vi "Online_Station.vi"(8 "error in (no error)":errorcluster, 11 "Main":T1={"Tite"="", "Base path"=path "", "Table"=[], "Stations"=[], "Shield Array"=[], "UPHs"=[], "VISA"={"VISA"="", "baud rate"=9600, "data bits"=8, "parity"=enum."None", "stop bits"=10, "flow control"=0}, "Path"={"roof"=path "", "Config"=path "", "Png"=path ""}, "Ctr"={"DB Dispaly"=refnum, "Error Table"=refnum, "Display"=refnum, "Login"=refnum, "Exit"=refnum, "FTT_Submit"=refnum}, "Login"={"User"="", "Grade"=""}, "information"={"cause"="", "Type"=enum."Inform", "code"=0, "Suroce"="", "Status"=FALSE}, "Local DB"={"Connstr"="", "Database"={"Constr"={"Driver"="", "Server"="", "User"="", "Pwd"="", "Database"=""}, "conn ref"=refnum, "State"=FALSE}}, "Remote DB"={"Connstr"="", "Database"={"Constr"={"Driver"="", "Server"="", "User"="", "Pwd"="", "Database"=""}, "conn ref"=refnum, "State"=FALSE}}, "FTT TV"="", "ExchangeTime"=0, "NVH"="", "EOL Path"=path ""} {"VISA"."flow control" items=["None", "XON/XOFF", "RTS/CTS", "XON/XOFF & RTS/CTS", "DTR/DSR", "XON/XOFF & DTR/DSR"]; "VISA"."stop bits" items=["1.0"=10, "1.5"=15, "2.0"=20]}) -> (0 "error out":errorcluster)   [LabVIEW 2014]
uses:
  Type'def/Online_Table.ctl
  <vilib>/ptbypt/NI_PtbyPt.lvlib
  Simatic S7/Function/Read/Read Sigle Data/Read Sigle String.vi
  <vilib>/addons/database/Connection.llb/Conn ObjectReference.ctl
  <vilib>/addons/database/NI_Database_API.lvlib
  Simatic S7/Function/Read/Read Sigle Data/Read Sigle Bool.vi
  Type'def/UPH Config.ctl
  VISA/Ctr/VISA Ctr.ctl
  Type'def/Main Ctr Ref.ctl
  Type'def/User Login.ctl
  Type'def/MainCtr.ctl
  Database/Ctr/Constr.ctl
  Database/Ctr/Conneect State.ctl
panel:
  out "Previous Event 2":string
  out "Previous Event":string
  in  "Test":bool
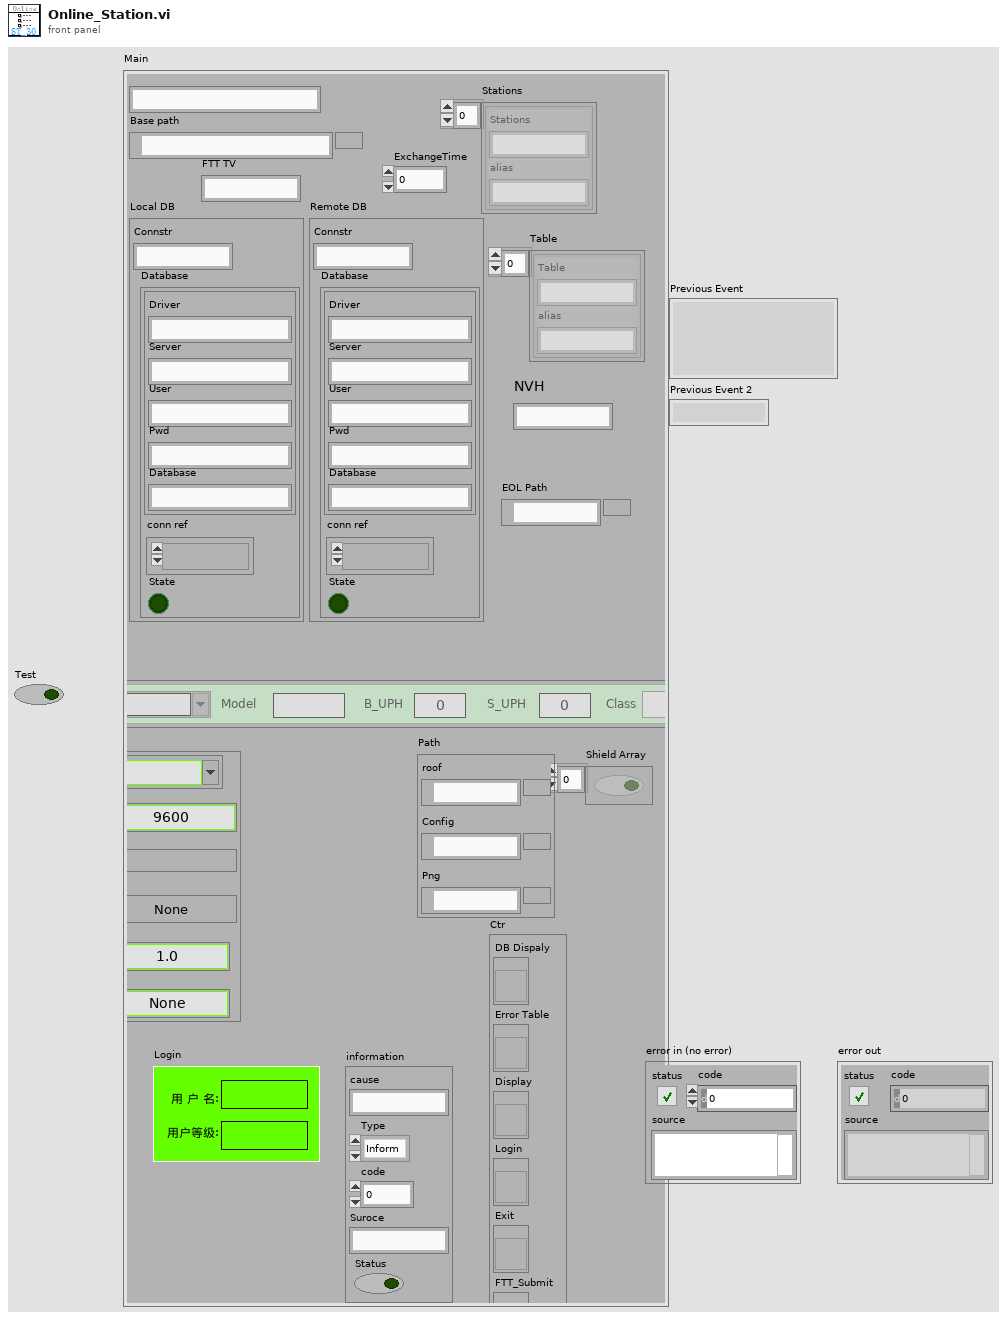
[diagram p1: front panel]
types:
  T1 = typedef "MainCtr.ctl" = cluster{"Tite":string, "Base path":path, "Table":cluster{"Table":string, "alias":string}[], "Stations":cluster{"Stations":string, "alias":string}[], "Shield Array":bool[], "UPHs":T2[], "VISA":T3, "Path":cluster{"roof":path, "Config":path, "Png":path}, "Ctr":T4, "Login":T5, "information":cluster{"cause":string, "Type":enum16{"Inform", "Warning", "Alarm"}, "code":i32, "Suroce":string, "Status":bool}, "Local DB":cluster{"Connstr":string, "Database":T6}, "Remote DB":cluster{"Connstr":string, "Database":T6}, "FTT TV":string, "ExchangeTime":i32, "NVH":string, "EOL Path":path}
  T2 = typedef "UPH Config.ctl" = cluster{"Line_No":string, "Model":string, "B_UPH ":i16, "S_UPH  ":i16, "Class":enum16{"Big", "Small"}}
  T3 = typedef "VISA Ctr.ctl" = cluster{"VISA":refnum<visa-resource-name>, "baud rate":u32, "data bits":u16, "parity":enum16{"None", "Odd", "Even", "Mark", "Space"}, "stop bits":u16, "flow control":u16}
  T4 = typedef "Main Ctr Ref.ctl" = cluster{"DB Dispaly":refnum<vi>, "Error Table":refnum<vi>, "Display":refnum<vi>, "Login":refnum<vi>, "Exit":refnum<vi>, "FTT_Submit":refnum<vi>}
  T5 = typedef "User Login.ctl" = cluster{"User":string, "Grade":string}
  T6 = typedef "Conneect State.ctl" = cluster{"Constr":T7, "conn ref":T8, "State":bool}
  T7 = typedef "Constr.ctl" = cluster{"Driver":string, "Server":string, "User":string, "Pwd":string, "Database":string}
  T8 = typedef "NI_Database_API.lvlib/Conn ObjectReference.ctl" = refnum<k1>
  T9 = cluster{"cause":string, "Type":enum16{"Inform", "Warning", "Alarm"}, "code":i32, "Suroce":string, "Status":bool}
  T10 = typedef "Online_Table.ctl" = cluster{"SN":string, "Frame":string, "Station":string, "Model":string, "Color":string, "OnTime":timestamp, "OutTime":timestamp, "Repaired":i32, "OnRepair":bool, "Pstate":string}
  T11 = cluster{"Main ":T1, "Online_Table":T10, "information":cluster{"cause":string, "Type":enum16{"Inform", "Warning", "Alarm"}, "code":i32, "Suroce":string, "Status":bool}, "ns":dbl}
  T12 = typedef "FTT Display Type.ctl" = cluster{"Line.No":string, "Model":string, "Color":string, "UPH":dbl, "Plan":dbl, "Target Rate":dbl, "Target ":dbl, "Actual":dbl, "FTT":dbl, "FTT Rate":dbl, "Repaired":dbl, "Reject":dbl, "Ouline":dbl, "Line State":string}
  T13 = cluster{"Display":T12, "Class":enum16{"Big", "Small"}}
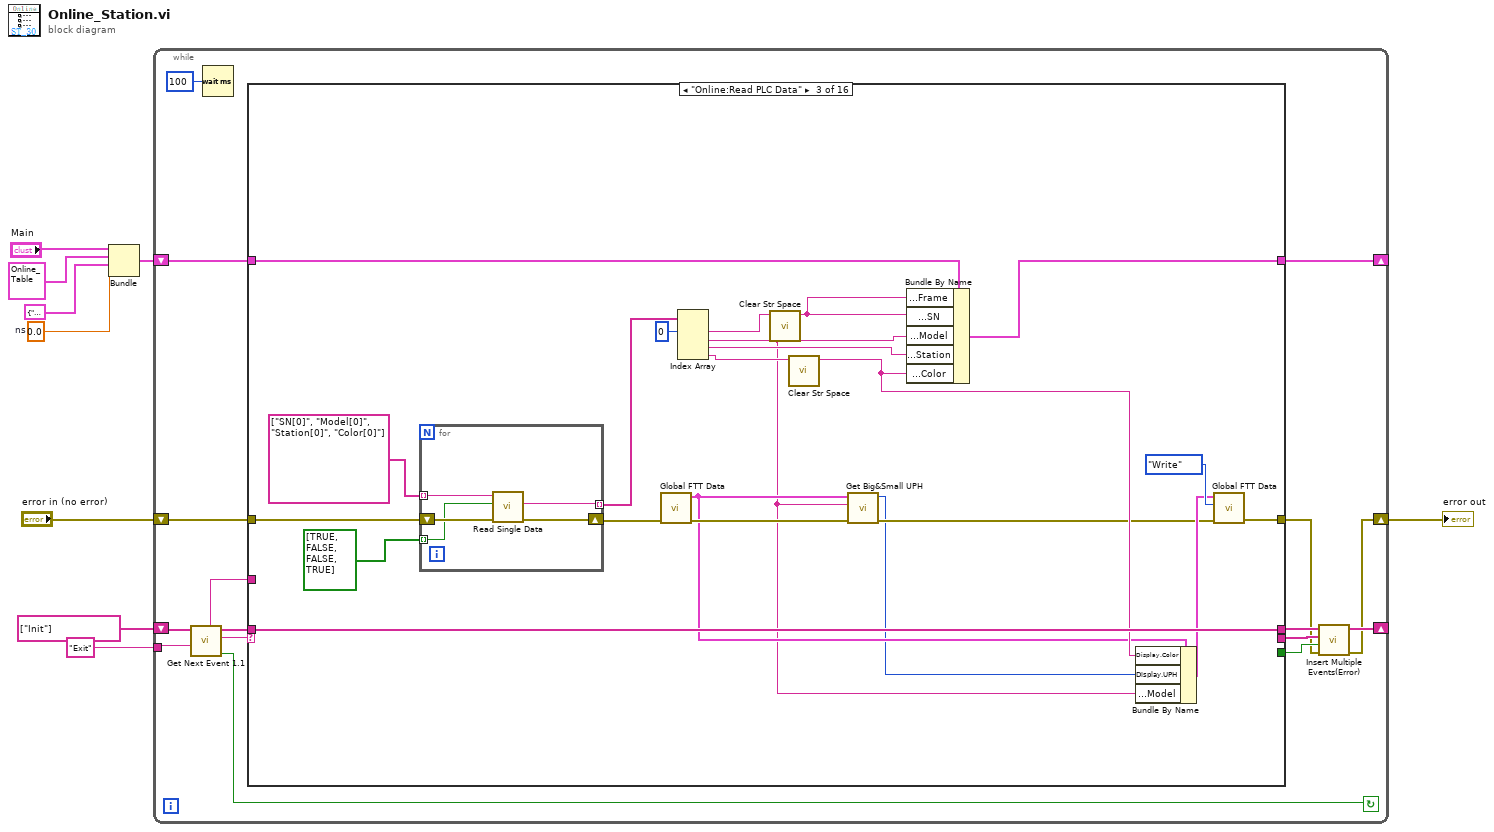
[diagram p0: block diagram]
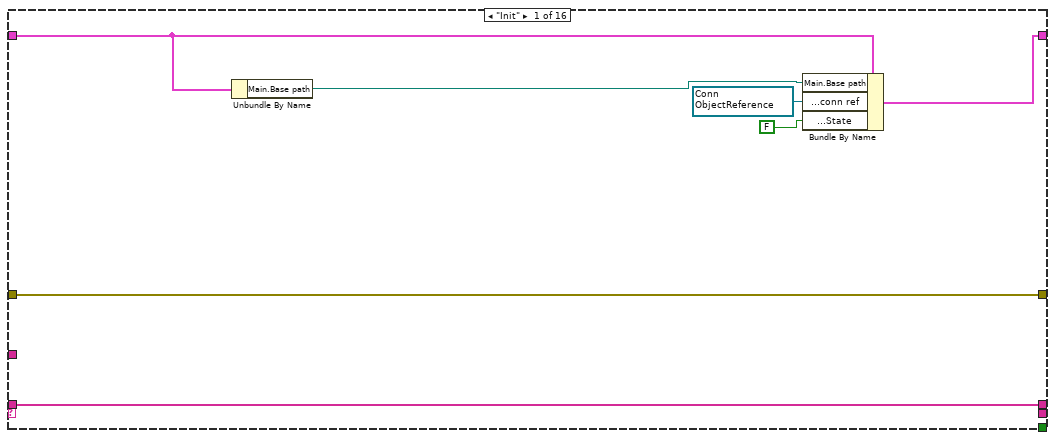
[diagram p2: hidden frame]
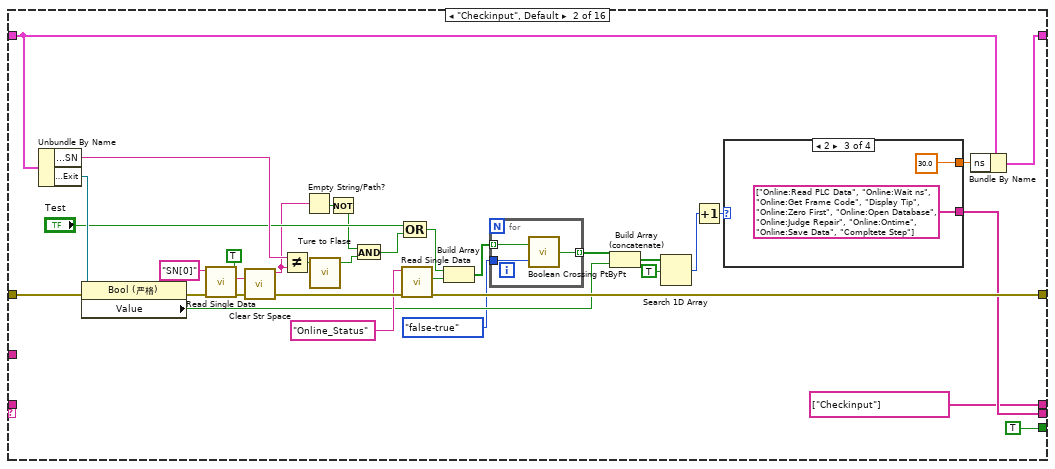
[diagram p3: hidden frame]
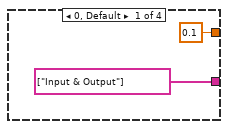
[diagram p4: hidden frame]
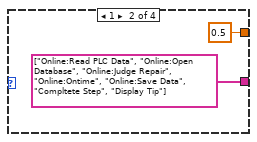
[diagram p5: hidden frame]
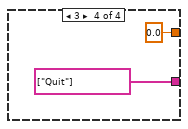
[diagram p6: hidden frame]
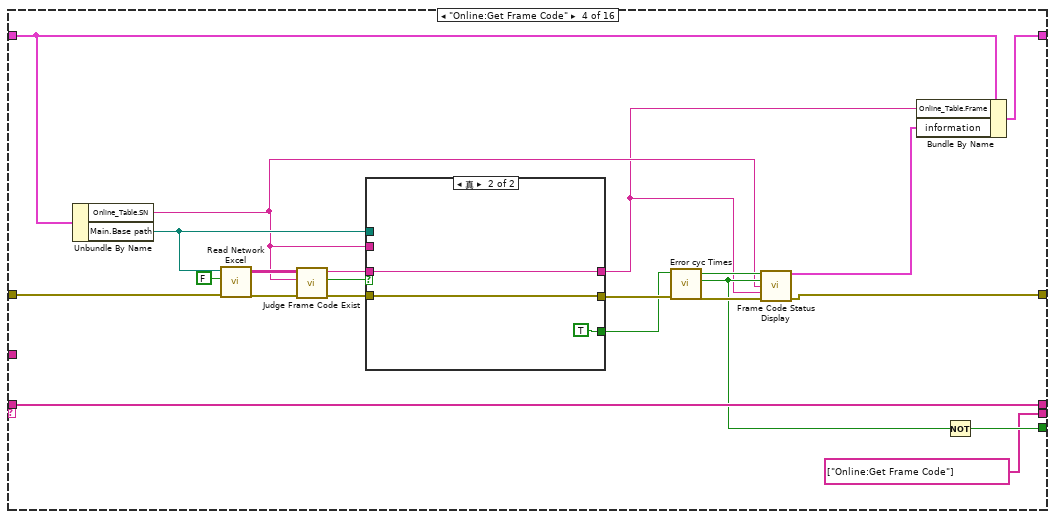
[diagram p7: hidden frame]
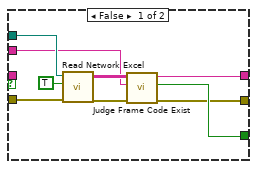
[diagram p8: hidden frame]
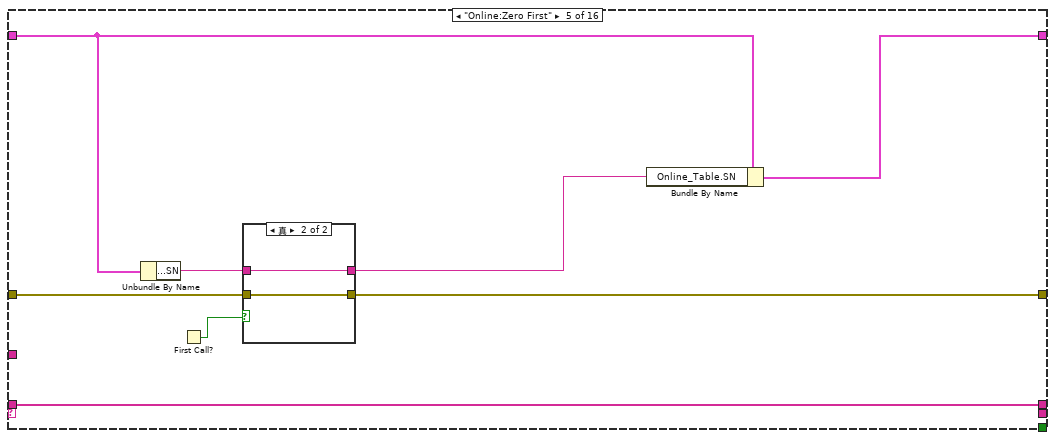
[diagram p9: hidden frame]
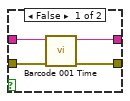
[diagram p10: hidden frame]
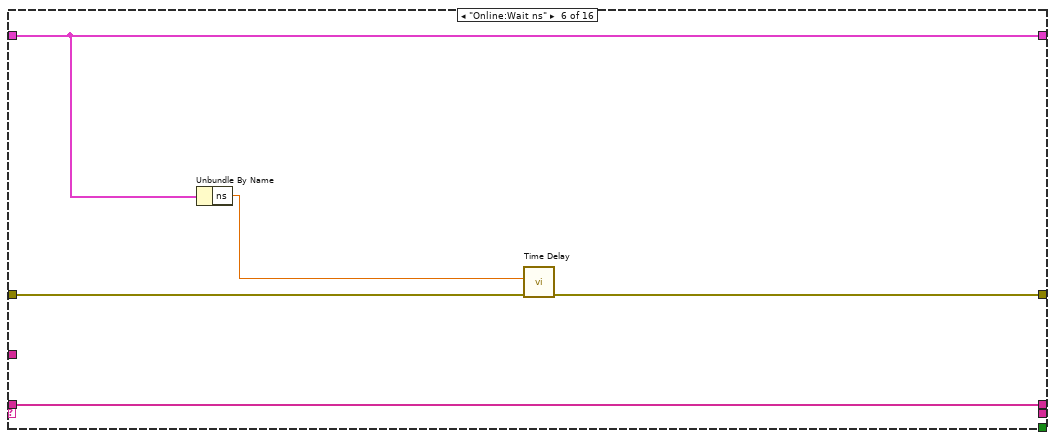
[diagram p11: hidden frame]
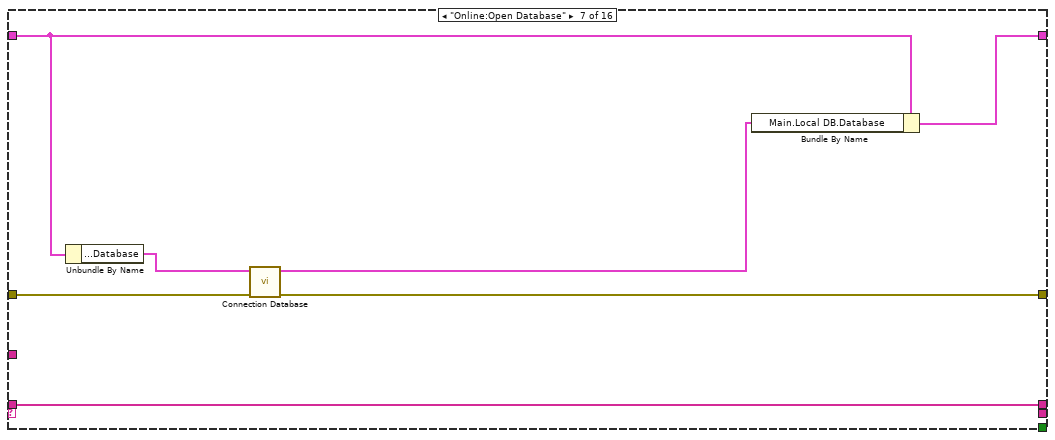
[diagram p12: hidden frame]
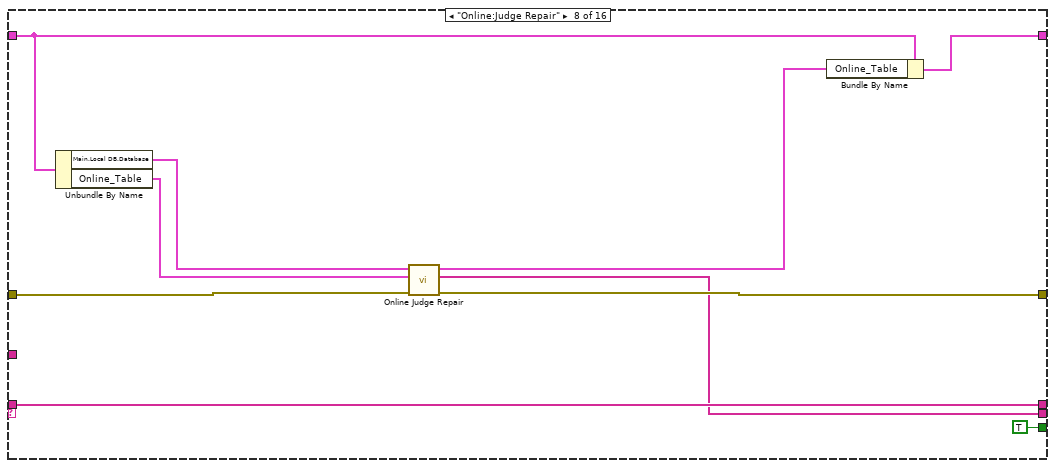
[diagram p13: hidden frame]
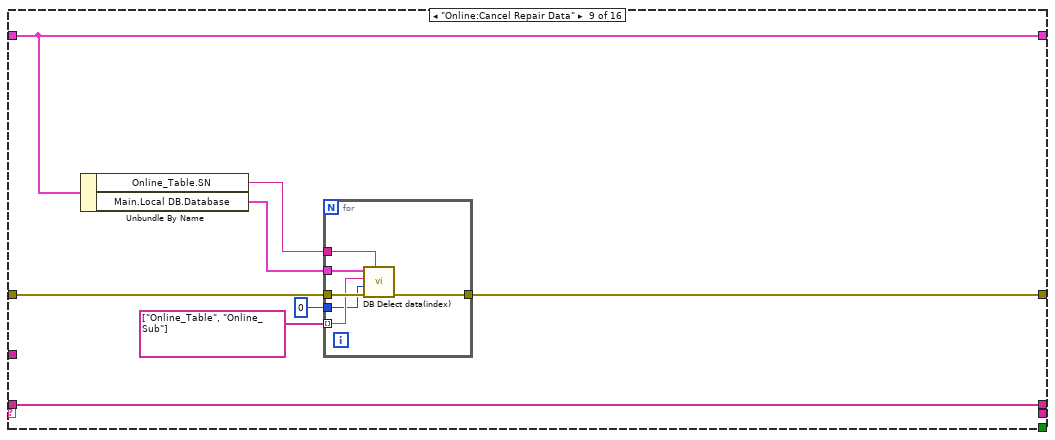
[diagram p14: hidden frame]
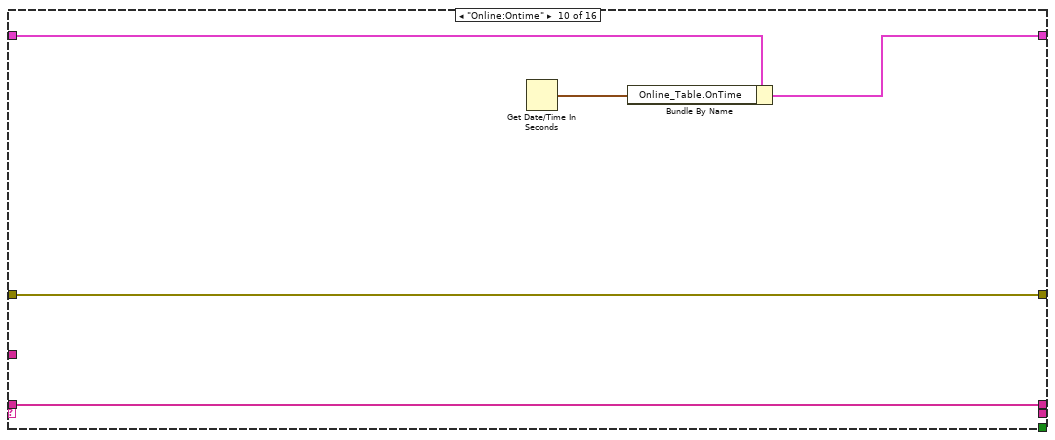
[diagram p15: hidden frame]
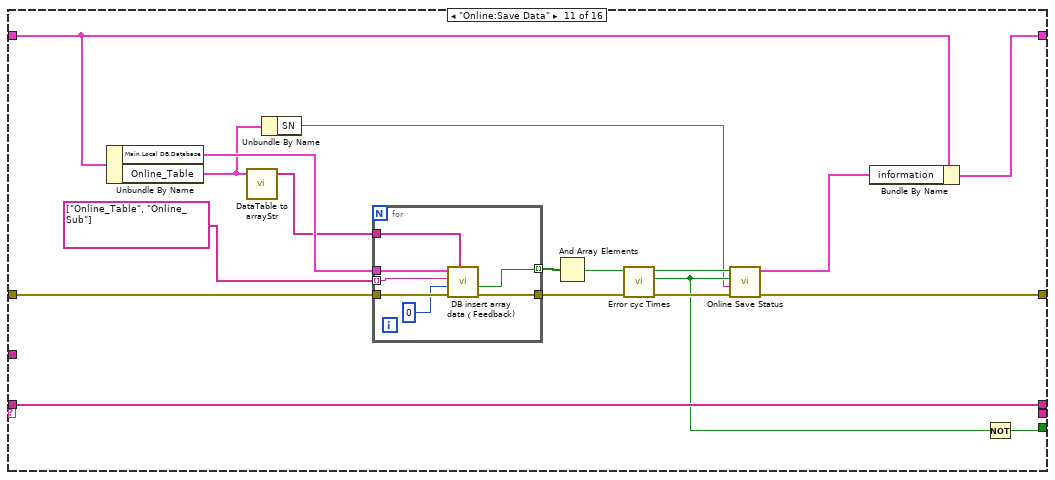
[diagram p16: hidden frame]
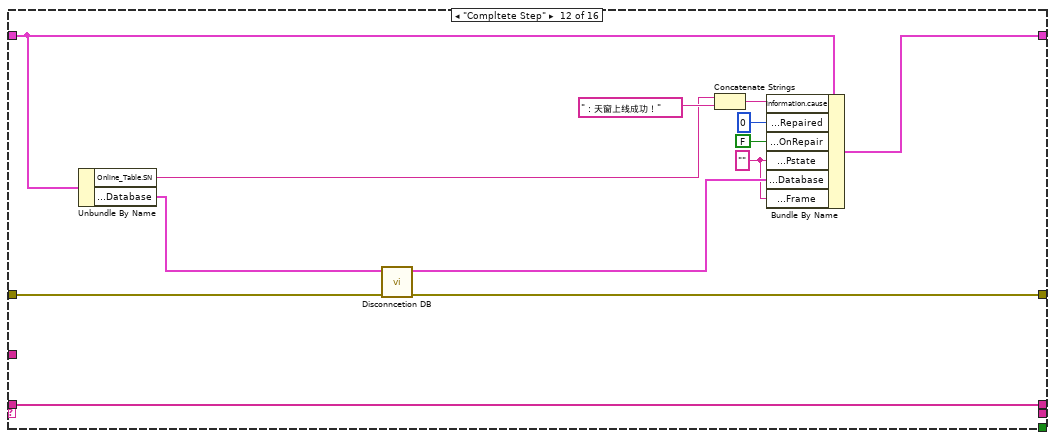
[diagram p17: hidden frame]
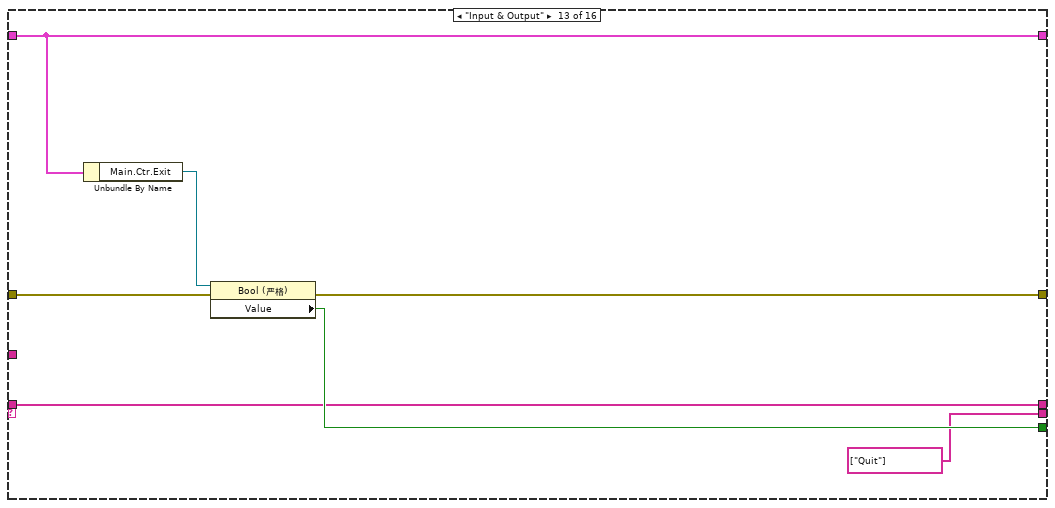
[diagram p18: hidden frame]
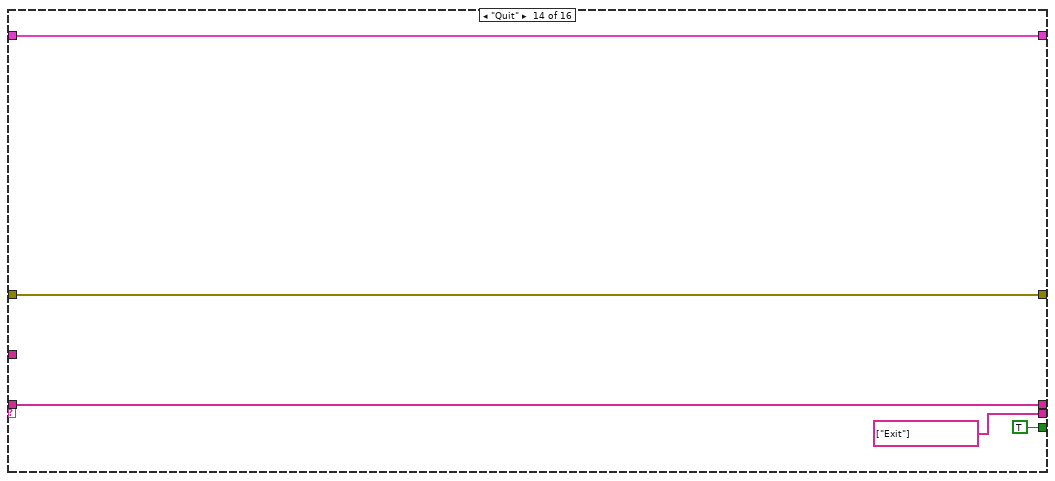
[diagram p19: hidden frame]
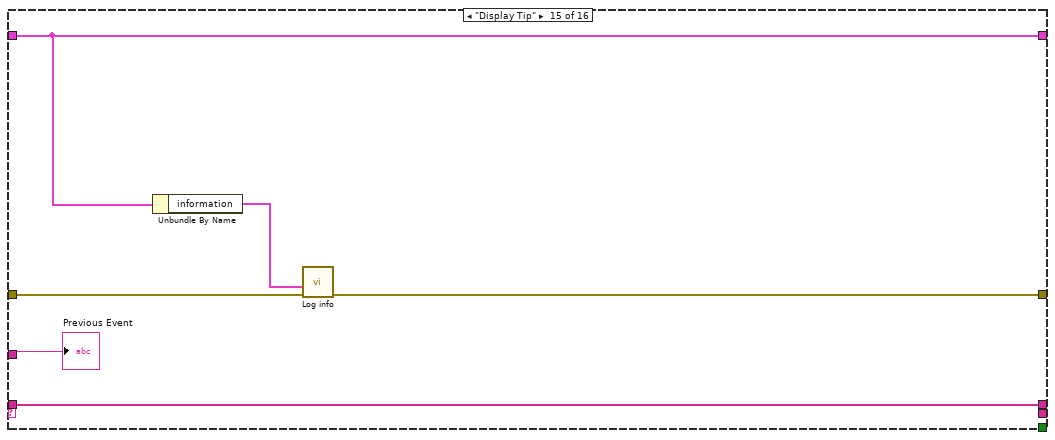
[diagram p20: hidden frame]
diagram:
  w1 = 0.0  # ns
  n1 = Bundle("Main"="Main", "Online_Table"=T10 {"SN"="", "Frame"="", "Station"="", "Model"="", "Color"="", "OnTime"=timestamp(0 s since 1904-01-01), "OutTime"=timestamp(0 s since 1904-01-01), "Repaired"=0, "OnRepair"=FALSE, "Pstate"=""}, "information"=T9 {"cause"="", "Type"=enum."Inform", "code"=0, "Suroce"="", "Status"=FALSE}, "ns"=w1) -> (w6:T11)  [unwired: 1 in]
  n2 = while {
    tunnel: "Exit" ("Exit Event") -> [w22]
    shift-right: [w18] -> _
    shift-left: string[] ["Init"] -> [w23]
    shift-right: [w12] -> w3
    shift-left: "error in (no error)" -> [w21]
    shift-right: [w14] -> _
    shift-left: w6 -> [w19]
    stop <- w24 continue-if-true
    n3 = call "Get Next Event 1.1.vi"("Exit Event"=w22, "event queue in"=w23) -> ("Condition (Exit:F)"=w24:bool, "next event"=w25:string, "event queue out"=w20:string[], "Previous Event"=w10:string)  [unwired: 6 in]
    n4 = Wait (ms)(milliseconds to wait=u32 100) -> ()  [unwired: 1 out]
    n5 = case shown="\"Online:Read PLC Data\"" w25 {
      tunnel: w21 -> [w31 w64 w98 w124 w144 w156 w160 w172 w179 w188 w209 w226 w236 w241 w248 w252]
      tunnel: w20 -> [w32 _ w94 w125 w142 w154 w163 w173 w181 w190 w210 w230 w232 w240 w244 _]
      tunnel: w19 -> [w29 w42 w96 w118 w141 w153 w162 w169 w180 w189 w194 w224 w237 w242 w246 w257]
      tunnel: [w31 w56 w88 w105 w143 w155 w158 w166 w174 w188 w200 w225 w234 w241 w247 w258] -> w13
      tunnel: [w32 string[] ["Checkinput"] w94 w125 w142 w154 w163 w173 w181 w190 w210 w230 w232 w240 w244 string[] ["Checkinput"]] -> w17
      tunnel: [_ TRUE ("Insert all? (T)") _ w113 _ _ _ TRUE ("Insert all? (T)") _ _ w202 _ w233 TRUE ("Insert all? (T)") _ FALSE ("Insert all? (T)")] -> w16
      tunnel: [_ w49 _ string[] ["Online:Get Frame Code"] _ _ _ w165 _ _ _ _ string[] ["Quit"] string[] ["Exit"] _ _] -> w15
      tunnel: [w30 w41 w95 w117 w140 w153 w161 w168 w180 w191 w193 w229 w237 w242 w246 w257] -> w14
      tunnel: w10 -> [_ _ _ _ _ _ _ _ _ _ _ _ _ _ w243 w250]
      frame "Init" {
        w27 = T8 refnum items=["Connection"] ("conn refer.conn ref")
        n6 = Unbundle By Name(w29) -> ("Main.Base path"=w28:path)
        n7 = Bundle By Name(cluster=w29, "Main.Base path"=w28, "Main.Local DB.Database.conn ref"=w27, "Main.Local DB.Database.State"=FALSE ("conn refer.State")) -> (w30:T11)
      }
      frame "Checkinput", Default {
        n8 = Unbundle By Name(w42) -> ("Online_Table.SN"=w61:string, "Main.Ctr.Exit"=w65:refnum<vi>)
        n9 = property class="Bool (严格)"(reference=w65, error in=w64) -> (error out=w63:errorcluster, "Value"=w55:bool)  [unwired: 1 out]
        n10 = call-poly "Read Single Data.vi"("error in (no error)"=w63, "Char/Str"=TRUE, "Tags"="SN[0]") -> ("error out"=w59:errorcluster, "Data Byte"=w39:string)  [unwired: 6 in, 1 out]
        n11 = call "Clear Str Space.vi"("SN"=w39) -> ("字符串"=w37:string)  [unwired: 10 in]
        n12 = Not Equal?(x=w61, y=w37) -> (x != y?=w60:bool)
        n13 = Empty String/Path?(string/path=w37) -> (empty?=w36:bool)
        n14 = call "Ture to Flase.vi"("in"=w60) -> ("Out"=w35:bool)  [unwired: 4 in]
        n15 = Not(x=w36) -> (.not. x?=w34:bool)
        n16 = And(x=w34, y=w35) -> (x .and. y?=w33:bool)
        n17 = call-poly "Read Single Data.vi"("error in (no error)"=w59, "Tags"="Online_Status") -> ("error out"=w56:errorcluster, "Boolean"=w46:bool)  [unwired: 7 in, 1 out]
        n18 = Compound Arithmetic op=OR("Test", w33) -> (w47:bool)
        n19 = Build Array(w47, w46) -> (w45:bool[])
        n20 = for {
          tunnel: w45 -> [w68] mode=indexing
          tunnel: enum16{"either", "false-true", "true-false"}."false-true" ("direction") -> [w67]
          tunnel: [w66] -> w43 mode=indexing
          n21 = call <vilib>:"Boolean Crossing PtByPt.vi"("direction"=w67, "input"=w68) -> ("crossing"=w66:bool)  [unwired: 1 in]
        }
        n22 = Build Array (concatenate)(w43, w55) -> (w54:bool[])
        n23 = Search 1D Array(1D array=w54, element=TRUE) -> (index of element=w52:i32)  [unwired: 1 in]
        n24 = Increment(x=w52) -> (x+1=w50:i32)
        n25 = case shown="2" w50 {
          tunnel: [string[] ["Input & Output"] string[] ["Online:Read PLC Data", "Online:Open Database", "Online:Judge Repair", "Online:Ontime", "Online:Save Data", "Compltete Step", "Display Tip"] string[] ["Online:Read PLC Data", "Online:Wait ns", "Online:Get Frame Code", "Display Tip", "Online:Zero First", "Online:Open Database", "Online:Judge Repair", "Online:Ontime", "Online:Save Data", "Compltete Step"] string[] ["Quit"]] -> w49
          tunnel: [0.1 0.5 30.0 0.0] -> w40
          frame 0, Default {
          }
          frame 1 {
          }
          frame 2 {
          }
          frame 3 {
          }
        }
        n26 = Bundle By Name(cluster=w42, "ns"=w40) -> (w41:T11)
      }
      frame "Online:Read PLC Data" {
        n27 = for {
          shift-right: [w102] -> w90
          shift-left: w98 -> [w103]
          tunnel: string[] ["SN[0]", "Model[0]", "Station[0]", "Color[0]"] -> [w101] mode=indexing
          tunnel: [w100] -> w93 mode=indexing
          tunnel: bool[] [TRUE, FALSE, FALSE, TRUE] -> [w99] mode=indexing
          n28 = call-poly "Read Single Data.vi"("error in (no error)"=w103, "Char/Str"=w99, "Tags"=w101) -> ("error out"=w102:errorcluster, "Data Byte"=w100:string)  [unwired: 6 in, 1 out]
        }
        n29 = call "Global FTT Data.vi"("error in (no error)"=w90) -> ("error out"=w81:errorcluster, "Cluster"=w80:T13)  [unwired: 9 in]
        n30 = Index Array(array=w93, index #1=0 ("index")) -> (element #1=w85:string, element #2=w79:string, element #3=w92:string, element #4=w83:string)  [unwired: 3 in]
        n31 = call "Clear Str Space.vi"("SN"=w85) -> ("字符串"=w84:string)  [unwired: 10 in]
        n32 = call "Clear Str Space.vi"("SN"=w83) -> ("字符串"=w82:string)  [unwired: 10 in]
        n33 = call "Get Big&Small UPH.vi"("error in (no error)"=w81, "Model"=w79, "Cluster"=w80) -> ("error out"=w78:errorcluster, "UPH"=w77:i16)  [unwired: 7 in]
        n34 = Bundle By Name(cluster=w96, "Online_Table.Frame"=w84, "Online_Table.SN"=w84, "Online_Table.Model"=w79, "Online_Table.Station"=w92, "Online_Table.Color"=w82) -> (w95:T11)
        n35 = Bundle By Name(cluster=w80, "Display.Color"=w82, "Display.UPH"=w77, "Display.Model"=w79) -> (w87:T13)
        n36 = call "Global FTT Data.vi"("error in (no error)"=w78, "Mode"=enum16{"Read", "Write"}."Write", "Display"=w87) -> ("error out"=w88:errorcluster)  [unwired: 7 in, 1 out]
      }
      frame "Online:Get Frame Code" {
        n37 = Unbundle By Name(w118) -> ("Online_Table.SN"=w108:string, "Main.Base path"=w116:path)
        n38 = call "Read Network Excel.vi"("error in (no error)"=w124, "T/Y"=FALSE, "Base Path"=w116) -> ("error out"=w123:errorcluster, "2DA_Str"=w122:string[][])  [unwired: 7 in]
        n39 = call "Judge Frame Code Exist.vi"("error in (no error)"=w123, "Online_Table.SN"=w108, "2DA_Str"=w122) -> ("error out"=w121:errorcluster, "Status"=w120:bool, "Frame Code"=w119:string)  [unwired: 6 in]
        n40 = case shown="真" w120 {
          tunnel: w121 -> [w133 w135]
          tunnel: w119 -> [_ w137]
          tunnel: [w127 w137] -> w107
          tunnel: w116 -> [w132 _]
          tunnel: w108 -> [w129 _]
          tunnel: [w128 TRUE ("Status")] -> w114
          tunnel: [w126 w135] -> w115
          frame False {
            n41 = call "Read Network Excel.vi"("error in (no error)"=w133, "T/Y"=TRUE, "Base Path"=w132) -> ("error out"=w134:errorcluster, "2DA_Str"=w130:string[][])  [unwired: 7 in]
            n42 = call "Judge Frame Code Exist.vi"("error in (no error)"=w134, "Online_Table.SN"=w129, "2DA_Str"=w130) -> ("error out"=w126:errorcluster, "Status"=w128:bool, "Frame Code"=w127:string)  [unwired: 6 in]
          }
          frame True {
          }
        }
        n43 = call "Error cyc Times.vi"("error in (no error)"=w115, "Status in"=w114) -> ("error out"=w111:errorcluster, "Cys Status"=w109:bool, "Status out"=w110:bool)  [unwired: 6 in, 1 out]
        n44 = call "Frame Code Status Display.vi"("Status"=w110, "Complete"=w109, "SN"=w108, "Frame"=w107, "error in (no error)"=w111) -> ("information"=w106:T9, "error out"=w105:errorcluster)  [unwired: 9 in]
        n45 = Bundle By Name(cluster=w118, "Online_Table.Frame"=w107, "information"=w106) -> (w117:T11)
        n46 = Not(x=w109) -> (.not. x?=w113:bool)
      }
      frame "Online:Zero First" {
        n47 = Unbundle By Name(w141) -> ("Online_Table.SN"=w145:string)
        n48 = First Call?() -> (First Call?: T/F=w138:bool)
        n49 = case shown="真" w138 {
          tunnel: w145 -> [w149 w150]
          tunnel: w144 -> [w148 w151]
          tunnel: [w147 w151] -> w143
          tunnel: [w146 w150] -> w139
          frame False {
            n50 = call "Barcode 001 Time.vi"("error in (no error)"=w148, "Code"=w149) -> ("error out"=w147:errorcluster, "Code out"=w146:string)  [unwired: 8 in]
          }
          frame True {
          }
        }
        n51 = Bundle By Name(cluster=w141, "Online_Table.SN"=w139) -> (w140:T11)
      }
      frame "Online:Wait ns" {
        n52 = Unbundle By Name(w153) -> ("ns"=w152:dbl)
        n53 = call "Time Delay"("error in (no error)"=w156, "Delay Time (s)"=w152) -> ("error out"=w155:errorcluster)  [unwired: 9 in]
      }
      frame "Online:Open Database" {
        n54 = Unbundle By Name(w162) -> ("Main.Local DB.Database"=w159:T6)
        n55 = call "Connection Database.vi"("error in (no error)"=w160, "Connncet State"=w159) -> ("error out"=w158:errorcluster, "Connncet State out"=w157:T6)  [unwired: 8 in]
        n56 = Bundle By Name(cluster=w162, "Main.Local DB.Database"=w157) -> (w161:T11)
      }
      frame "Online:Judge Repair" {
        n57 = Unbundle By Name(w169) -> ("Main.Local DB.Database"=w171:T6, "Online_Table"=w170:T10)
        n58 = call "Online Judge Repair.vi"("error in (no error)"=w172, "Online_Table"=w170, "conn refer"=w171) -> ("error out"=w166:errorcluster, "Steps"=w165:string[], "Online_Table out"=w167:T10)  [unwired: 6 in]
        n59 = Bundle By Name(cluster=w169, "Online_Table"=w167) -> (w168:T11)
      }
      frame "Online:Cancel Repair Data" {
        n60 = Unbundle By Name(w180) -> ("Online_Table.SN"=w175:string, "Main.Local DB.Database"=w178:T6)
        n61 = for {
          tunnel: w179 -> [w187]
          tunnel: w178 -> [w186]
          tunnel: string[] ["Online_Table", "Online_Sub"] -> [w185] mode=indexing
          tunnel: 0 ("index") -> [w184]
          tunnel: w175 -> [w183]
          tunnel: [w182] -> w174
          n62 = call "DB Delect data(index).vi"("code"=w183, "error in (no error)"=w187, "index"=w184, "table"=w185, "Connncet State"=w186) -> ("error out"=w182:errorcluster)  [unwired: 4 in, 2 out]
        }
      }
      frame "Online:Ontime" {
        n63 = Get Date/Time In Seconds() -> (seconds since 1Jan1904=w192:timestamp)
        n64 = Bundle By Name(cluster=w189, "Online_Table.OnTime"=w192) -> (w191:T11)
      }
      frame "Online:Save Data" {
        n65 = Unbundle By Name(w194) -> ("Main.Local DB.Database"=w208:T6, "Online_Table"=w197:T10)
        n66 = call "DataTable to arrayStr.vi"("Online_Table"=w197) -> ("appended array"=w206:string[])  [unwired: 4 in]
        n67 = Unbundle By Name(w197) -> ("SN"=w196:string)
        n68 = for {
          tunnel: w209 -> [w217]
          tunnel: w208 -> [w216]
          tunnel: string[] ["Online_Table", "Online_Sub"] -> [w215] mode=indexing
          tunnel: [w213] -> w204
          tunnel: w206 -> [w212]
          tunnel: [w211] -> w205 mode=indexing
          n69 = call "DB insert array data（Feedback).vi"("Data"=w212, "error in (no error)"=w217, "index"=0, "table"=w215, "Connncet State"=w216) -> ("error out"=w213:errorcluster, "state"=w211:bool)  [unwired: 4 in, 1 out]
        }
        n70 = And Array Elements(Boolean array=w205) -> (logical AND=w203:bool)
        n71 = call "Error cyc Times.vi"("error in (no error)"=w204, "Status in"=w203) -> ("error out"=w201:errorcluster, "Cys Status"=w198:bool, "Status out"=w199:bool)  [unwired: 6 in, 1 out]
        n72 = call "Online Save Status.vi"("error in (no error)"=w201, "SN"=w196, "Complete"=w198, "Status"=w199) -> ("error out"=w200:errorcluster, "information"=w195:T9)  [unwired: 6 in]
        n73 = Bundle By Name(cluster=w194, "information"=w195) -> (w193:T11)
        n74 = Not(x=w198) -> (.not. x?=w202:bool)
      }
      frame "Compltete Step" {
        w218 = "" ("Online_Table.Pstate")
        n75 = Unbundle By Name(w224) -> ("Online_Table.SN"=w220:string, "Main.Local DB.Database"=w223:T6)
        n76 = call "Disconncetion DB.vi"("error in (no error)"=w226, "Connncet State"=w223) -> ("error out"=w225:errorcluster, "Connect State"=w219:T6)  [unwired: 8 in]
        n77 = Concatenate Strings(w220, "：天窗上线成功！" ("information.cause")) -> (w222:string)
        n78 = Bundle By Name(cluster=w224, "information.cause"=w222, "Online_Table.Repaired"=0, "Online_Table.OnRepair"=FALSE, "Online_Table.Pstate"=w218, "Main.Local DB.Database"=w219, "Online_Table.Frame"=w218) -> (w229:T11)
      }
      frame "Input & Output" {
        n79 = Unbundle By Name(w237) -> ("Main.Ctr.Exit"=w235:refnum<vi>)
        n80 = property class="Bool (严格)"(reference=w235, error in=w236) -> (error out=w234:errorcluster, "Value"=w233:bool)  [unwired: 1 out]
      }
      frame "Quit" {
      }
      frame "Display Tip" {
        n81 = Unbundle By Name(w246) -> ("information"=w245:T9)
        n82 = call "Log info.vi"("error in (no error)"=w248, "information"=w245) -> ("error out"=w247:errorcluster)  [unwired: 8 in, 1 out]
        "Previous Event" <- w243
      }
      frame "Error Log" {
        n83 = Unbundle By Name(w257) -> ("information"=w256:T9)
        n84 = Unbundle By Name(w252) -> ("source"=w251:string)
        n85 = Bundle By Name(cluster=w256, "Status"=TRUE, "cause"=w251) -> (w255:T9)
        n86 = call "Log info.vi"("error in (no error)"=w252, "information"=w255) -> ("error out"=w259:errorcluster)  [unwired: 8 in, 1 out]
        n87 = call <vilib>:"Clear Errors.vi"("error in (no error)"=w259) -> ("error out"=w258:errorcluster)  [unwired: 5 in, 1 out]
        "Previous Event 2" <- w250
      }
    }
    n88 = call "Insert Multiple Events(Error).vi"("error in (no error)"=w13, "Insert all? (T)"=w16, "Events to Insert"=w15, "Event queue in"=w17) -> ("error out"=w12:errorcluster, "Event queue out"=w18:string[])  [unwired: 6 in]
  }
  "error out" <- w3
